vi "MeasurementCluster.vi"() -> ()   [LabVIEW 2017]
panel:
  in  "MeasurementCluster":T1
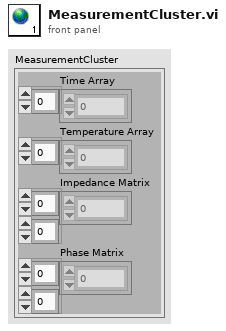
[diagram p1: front panel]
types:
  T1 = cluster{"Impedance Matrix":dbl[][], "Phase Matrix":dbl[][], "Time Array":dbl[], "Temperature Array":dbl[]}
diagram:
